vi "NanotecSMCPDDriver.set rotation direction.vi"(0 "VISA resource name":refnum<visa-resource-name>, 1 "contollerID":i32=-1, 3 "clock-wise":bool, 5 "error in (no error)":errorcluster) -> (14 "VISA resource name out":refnum<visa-resource-name>, 15 "contollerID out":i32=-1, 19 "error out":errorcluster)   [LabVIEW 2014, in "NanotecSMCPDDriver.lvlib"]
doc: "Sets the direction of turning for a relative movement."
uses:
  NanotecSMCPDDriver.lvlib
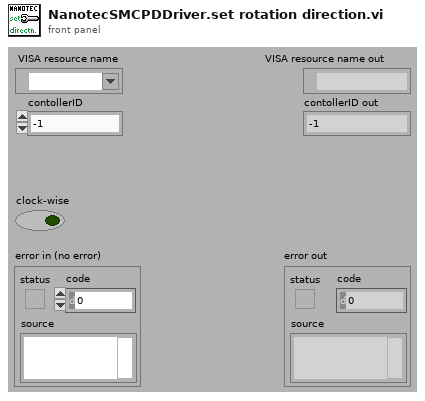
[diagram p1: front panel]
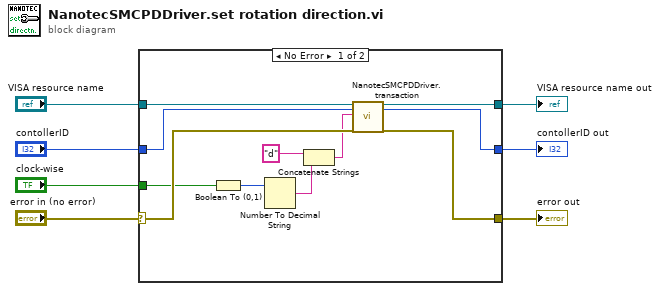
[diagram p0: block diagram]
diagram:
  n1 = case shown="No Error" "error in (no error)" {
    selector: "error in (no error)" -> [w13 w19]
    tunnel: [w17 w21] -> w7
    tunnel: [w16 w19] -> w6
    tunnel: "VISA resource name" -> [w15 w21]
    tunnel: "contollerID" -> [w14 w20]
    tunnel: [w18 w20] -> w3
    tunnel: "clock-wise" -> [w8 _]
    frame No Error {
      n2 = Boolean To (0,1)(Boolean=w8) -> (0, 1=w9:i16)
      n3 = Number To Decimal String(number=w9) -> (decimal integer string=w12:string)  [unwired: 1 in]
      n4 = Concatenate Strings("d" ("commandString"), w12) -> (w10:string)
      n5 = call "NanotecSMCPDDriver.transaction.vi"("VISAresource"=w15, "contollerID"=w14, "commandString"=w10, "error in (no error)"=w13) -> ("VISAresource out"=w17:refnum<visa-resource-name>, "contollerID out"=w18:i32, "error out"=w16:errorcluster)  [unwired: 10 in, 3 out]
    }
    frame Error {
    }
  }
  "VISA resource name out" <- w7
  "error out" <- w6
  "contollerID out" <- w3
